vi "NI VISA Write .vi"() -> ()   [LabVIEW 2016]
panel:
  in  "green":bool
  in  "red":bool
  in  "stop":bool
  out "red no.":dbl
  out "green no.":dbl
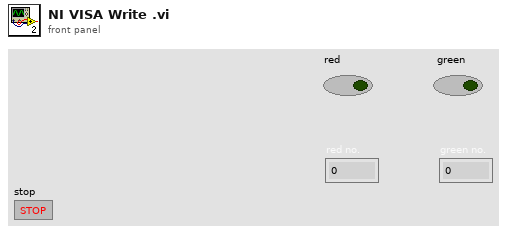
[diagram p1: front panel]
types:
  T1 = enum16{"Read", "Write", "ReadWrite", "BufferedRead", "BufferedReadWrite"}
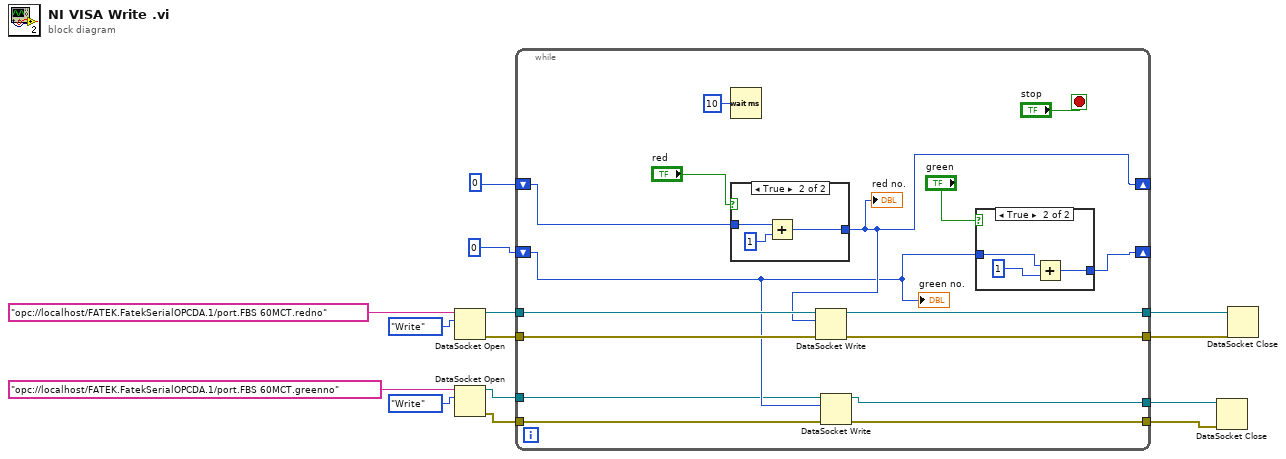
[diagram p0: block diagram]
diagram:
  n1 = DataSocket Open(10:T1."Write" ("mode"), 11:"opc://localhost/FATEK.FatekSerialOPCDA.1/port.FBS 60MCT.redno") -> (0:w11:errorcluster, 3:w12:refnum<k13>)  [unwired: 2 in]
  n2 = DataSocket Open(10:T1."Write" ("mode"), 11:"opc://localhost/FATEK.FatekSerialOPCDA.1/port.FBS 60MCT.greenno") -> (0:w3:errorcluster, 3:w4:refnum<k13>)  [unwired: 2 in]
  n3 = while {
    shift-right: [w23] -> _
    shift-left: 0 -> [w29]
    shift-right: [w28] -> _
    shift-left: 0 -> [w19]
    tunnel: w12 -> [w27]
    tunnel: w11 -> [w26]
    tunnel: [w25] -> w10
    tunnel: [w24] -> w9
    tunnel: w4 -> [w18]
    tunnel: w3 -> [w17]
    tunnel: [w16] -> w2
    tunnel: [w15] -> w1
    stop <- "stop" stop-if-true
    n4 = Wait (ms)(milliseconds to wait=u32 10) -> ()  [unwired: 1 out]
    n5 = case shown="True" "red" {
      tunnel: w29 -> [w31 w34]
      tunnel: [w31 w33] -> w23
      frame False {
      }
      frame True {
        n6 = Add(x=w34, y=1) -> (x+y=w33:i32)
      }
    }
    "red no." <- w23
    n7 = DataSocket Write(8:w26, 10:w23, 11:w27) -> (0:w24:errorcluster, 3:w25:refnum<k13>)  [unwired: 1 in, 1 out]
    n8 = DataSocket Write(8:w17, 10:w19, 11:w18) -> (0:w15:errorcluster, 3:w16:refnum<k13>)  [unwired: 1 in, 1 out]
    n9 = case shown="True" "green" {
      tunnel: [w35 w38] -> w28
      tunnel: w19 -> [w35 w37]
      frame False {
      }
      frame True {
        n10 = Add(x=w37, y=1) -> (x+y=w38:i32)
      }
    }
    "green no." <- w19
  }
  n11 = DataSocket Close(8:w1, 11:w2) -> ()  [unwired: 1 in, 2 out]
  n12 = DataSocket Close(8:w9, 11:w10) -> ()  [unwired: 1 in, 2 out]
